vi "Teleop.vi"(10 "Match Info":T1={"Autonomous Elapsed Seconds"=0.0, "TeleOp Elapsed Seconds"=0.0, "Disabled Elapsed Seconds"=0.0, "Visited Autonomous"=FALSE, "Visited TeleOp"=FALSE, "Visited Disabled"=FALSE, "Autonomous Settings"={"Autonomous Style"=enum."Independent", "VI Refnum"=refnum}}, 11 "Call Context":T2) -> ()   [LabVIEW 2018]
doc: "This VI is called for each TeleOp packet received from the DS where the robot is not disabled. It is often used to read from the joysticks and update I/O or to update setpoints for timed control loops. It should complete and return within 20 milliseconds or it may miss DS packets."
uses:
  <vilib>/ptbypt/NI_PtbyPt.lvlib
  <vilib>/addons/control/pid/NI_PID_pid.lvlib
  <vilib>/addons/control/pid/pid.llb/PID Output Rate Limiter (DBL).vi
  <vilib>/Rock Robotics/Network Tables/NT Write Number.vi
  Robot Global Data.vi
  <vilib>/Rock Robotics/Network Tables/NT Write String.vi
  <vilib>/Rock Robotics/Network Tables/NT Write Numeric Array.vi
  <vilib>/Rock Robotics/WPI/DriverStation/WPI_DriverStationMatch Info.ctl
  <vilib>/Rock Robotics/WPI/DriverStation/WPI_DriverStationDerivedRobotMode.ctl
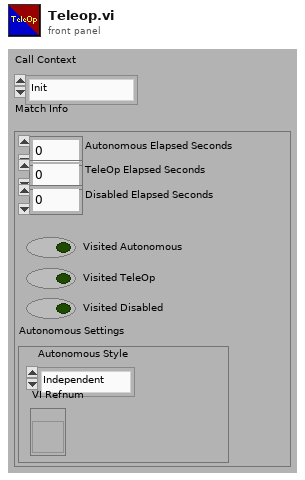
[diagram p1: front panel]
types:
  T1 = typedef "WPI_DriverStationMatch Info.ctl" = cluster{"Autonomous Elapsed Seconds":dbl, "TeleOp Elapsed Seconds":dbl, "Disabled Elapsed Seconds":dbl, "Visited Autonomous":bool, "Visited TeleOp":bool, "Visited Disabled":bool, "Autonomous Settings":cluster{"Autonomous Style":enum16{"Iterative", "Independent"}, "VI Refnum":refnum<vi>}}
  T2 = typedef "WPI_DriverStationDerivedRobotMode.ctl" = enum16{"Init", "Execute", "Stop"}
  T3 = cluster{void, "Filtered x":dbl, "mean":dbl, "output":dbl}
  T4 = typedef "WPI_AnalogChannelDevRef.ctl" = cluster{"DevStatus":errorcluster, "Analog Channel":T5}
  T5 = typedef "FPGA_AIChannel.ctl" = enum8{"AI 0", "AI 1", "AI 2", "AI 3", "AI MXP 0", "AI MXP 1", "AI MXP 2", "AI MXP 3", "Invalid"}
  T6 = typedef "WPI_JoystickDevRef.ctl" = cluster{"Device":T7}
  T7 = typedef "WPI_JoystickDeviceEnum.ctl" = enum16{"USB 0", "USB 1", "USB 2", "USB 3", "USB 4", "USB 5"}
  T8 = typedef "WPI_RobotDriveDevRef.ctl" = cluster{"DevStatus":errorcluster, "Motors[]":T9[], "Square Inputs":bool, "Max Output":dbl}
  T9 = typedef "WPI_MotorControlDeviceRef.ctl" = cluster{"DeviceStatus":errorcluster, "Type":T10, "PWM":cluster{"PWM Channel":T11, "DeadBand":T12}, "CAN":cluster{"Device Number":u8, "SetOutput VI Ref":variant, "GetOutput VI Ref":variant, "Enable VI Ref":variant, "Disable VI Ref":variant, "Data":variant}, "Invert":bool, "DIO PWM":cluster{"PWM \"Enable\" Channel":T11, "DIOChannel":T13, "PWM Rate":dbl}}
  T10 = typedef "WPI_MotorControlType.ctl" = enum16{"PWM", "CAN", "DIO PWM"}
  T11 = typedef "FPGA_DIOPWMChannel.ctl" = enum8{"PWM 0", "PWM 1", "PWM 2", "PWM 3", "PWM 4", "PWM 5", "PWM 6", "PWM 7", "PWM 8", "PWM 9", "PWM MXP 0", "PWM MXP 1", "PWM MXP 2", "PWM MXP 3", "PWM MXP 4", "PWM MXP 5", "PWM MXP 6", "PWM MXP 7", "PWM MXP 8", "PWM MXP 9", "Invalid"}
  T12 = typedef "WPI_PWMDeadband.ctl" = cluster{"Name":string, "maxPositivePwm":i32, "minPositivePwm":i32, "centerPwm":i32, "maxNegativePwm":i32, "minNegativePwm":i32, "angularRange":u16}
  T13 = typedef "FPGA_DIOChannel.ctl" = enum8{"DIO 0", "DIO 1", "DIO 2", "DIO 3", "DIO 4", "DIO 5", "DIO 6", "DIO 7", "DIO 8", "DIO 9", "DIO MXP 0", "DIO MXP 1", "DIO MXP 2", "DIO MXP 3", "DIO MXP 4", "DIO MXP 5", "DIO MXP 6", "DIO MXP 7", "DIO MXP 8", "DIO MXP 9", "DIO MXP 10", "DIO MXP 11", "DIO MXP 12", "DIO MXP 13", "DIO MXP 14", "DIO MXP 15", "SPI Port CS1", "SPI Port CS2", "SPI Port CS3", "SPI Port MISO", "SPI Port MOSI", "Invalid"}
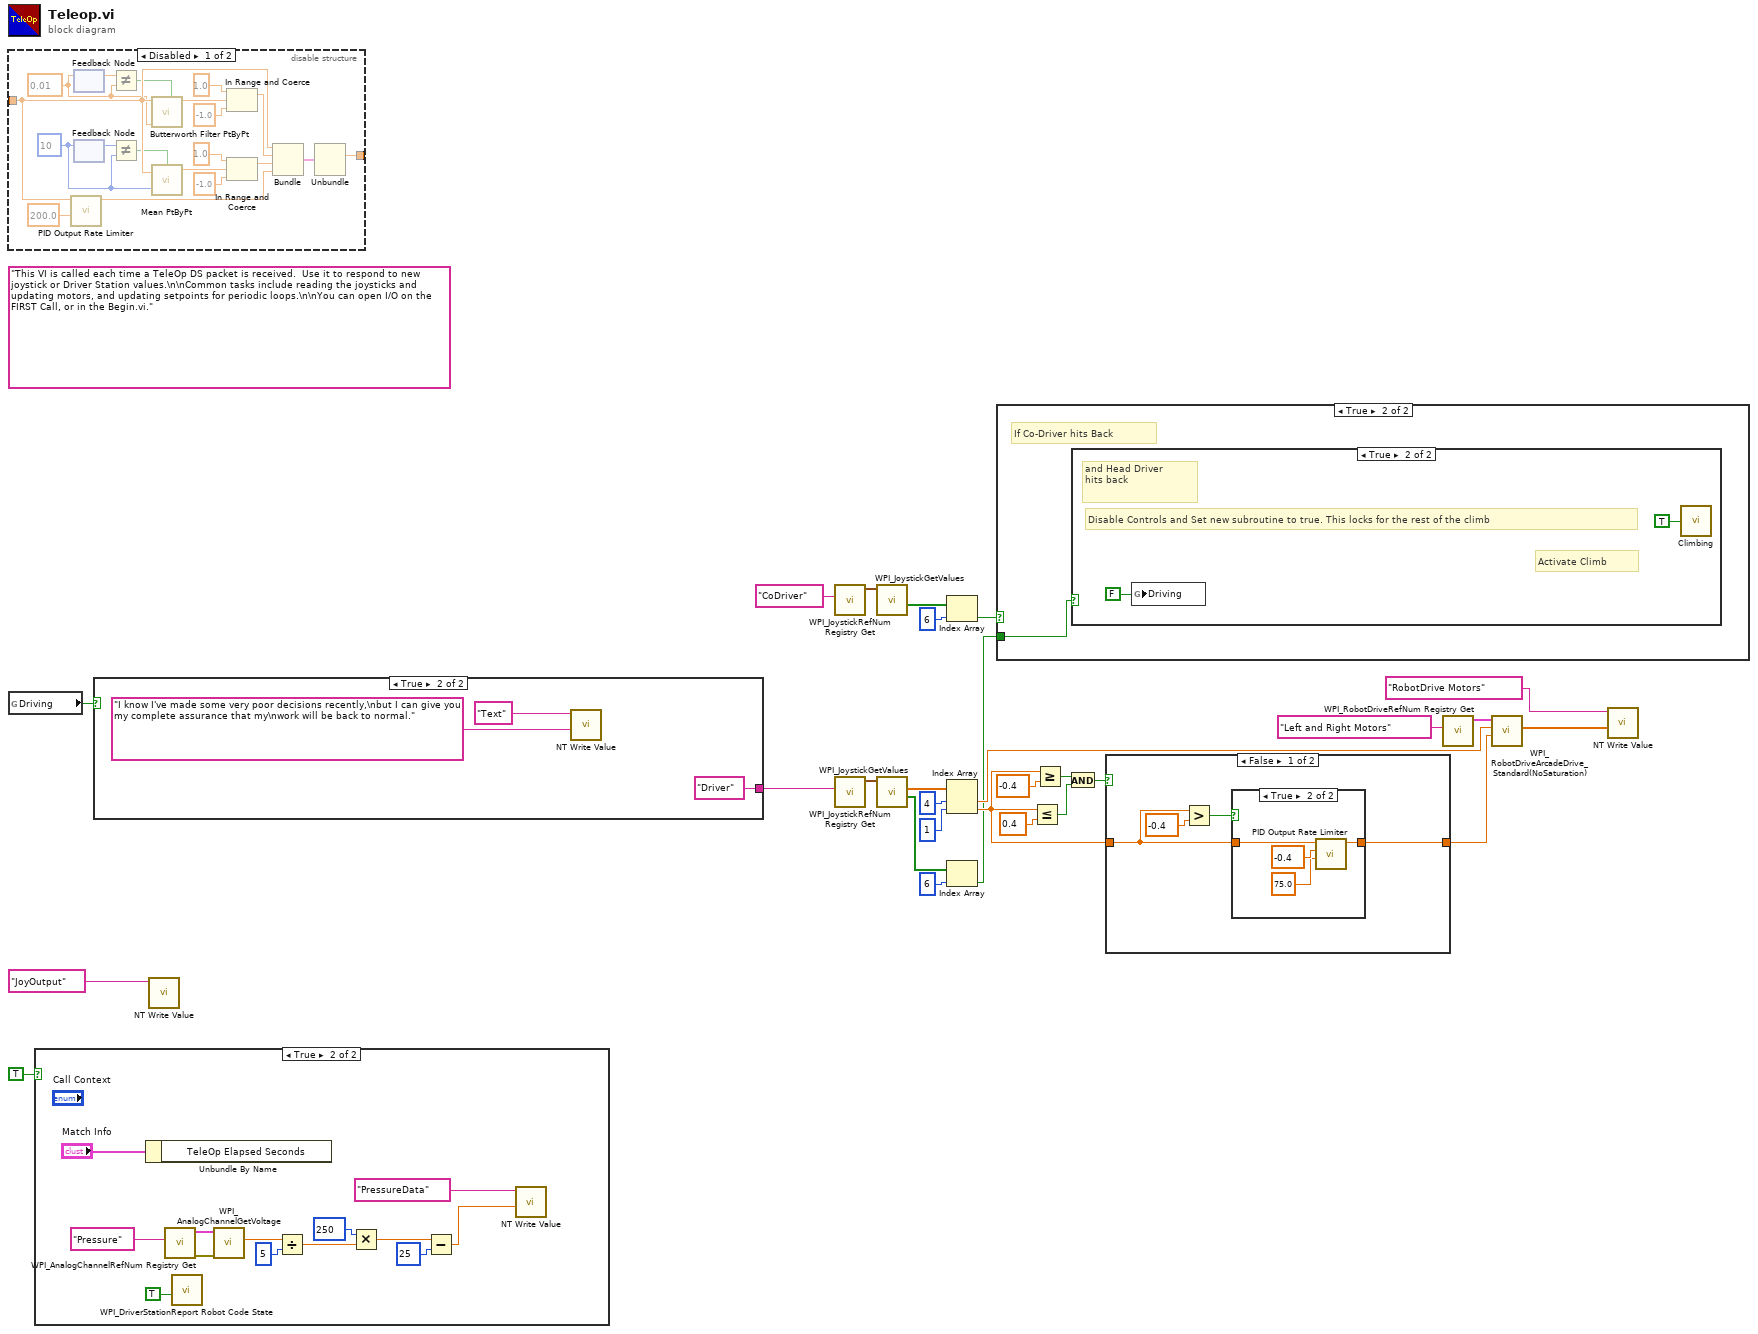
[diagram p0: block diagram]
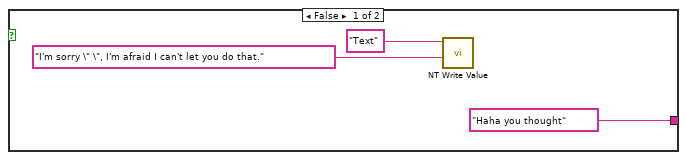
[diagram p5: hidden frame]
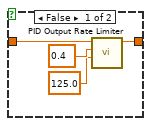
[diagram p6: hidden frame]
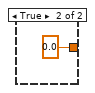
[diagram p7: hidden frame]
diagram:
  (unwired) "This VI is called each time a TeleOp DS packet is received.  Use it to respond to new joystick or Driver Station values.\n\nCommon tasks include reading the joysticks and updating motors, and updating setpoints for periodic loops.\n\nYou can open I/O on the FIRST Call, or in the Begin.vi."
  n1 = disable-structure shown="Disabled" {
    disable-tunnel: _ -> [w47 _]
    disable-tunnel: [w29 _] -> _
    frame Disabled {
      w39 = 10
      w45 = 0.01
      n2 = call-poly <vilib>:"PID Output Rate Limiter.vi"("output rate (EGU/min)"=200.0, "input (controller output)"=w47) -> ("output"=w31:dbl)  [unwired: 6 in, 1 out]
      n3 = feedback #1() -> (w46:dbl)  [unwired: 1 in]
      n4 = feedback-in #1(w45) -> ()
      n5 = feedback #2() -> (w40:i32)  [unwired: 1 in]
      n6 = feedback-in #2(w39) -> ()
      n7 = Not Equal?(x=w46, y=w45) -> (x != y?=w44:bool)
      n8 = Not Equal?(x=w40, y=w39) -> (x != y?=w38:bool)
      n9 = call <vilib>:"Butterworth Filter PtByPt.vi"("initialize"=w44, "low cutoff freq: fl"=w45, "x"=w47) -> ("Filtered x"=w43:dbl)  [unwired: 6 in, 1 out]
      n10 = call <vilib>:"Mean PtByPt.vi"("x"=w47, "sample length"=w39, "initialize"=w38) -> ("mean"=w35:dbl)  [unwired: 1 in, 1 out]
      n11 = In Range and Coerce(upper limit=1.0, x=w43, lower limit=-1.0) -> (coerced(x)=w33:dbl)  [unwired: 1 out]
      n12 = In Range and Coerce(upper limit=1.0, x=w35, lower limit=-1.0) -> (coerced(x)=w32:dbl)  [unwired: 1 out]
      n13 = Bundle(w47, "Filtered x"=w33, "mean"=w32, "output"=w31) -> (w30:T3)  [unwired: 1 in]
      n14 = Unbundle(w30) -> ("Filtered x"=w29:dbl)  [unwired: 3 out]
    }
    frame Enabled {
    }
  }
  n15 = global read "Robot Global Data.vi" "Driving"() -> (w11:bool)
  n16 = case shown="True" TRUE {
    frame False {
    }
    frame True {
      n17 = Unbundle By Name("Match Info") -> ()  [unwired: 1 out]
      n18 = call <vilib>:"WPI_AnalogChannelRefNum Registry Get.vi"("refnum name"="Pressure") -> ("error out"=w57:errorcluster, "AIDeviceRef"=w56:T4)  [unwired: 9 in]
      n19 = call <vilib>:"WPI_DriverStationReport Robot Code State.vi"("TeleOp"=TRUE ("Autonomous")) -> ()  [unwired: 10 in, 1 out]
      n20 = call <vilib>:"WPI_AnalogChannelGetVoltage.vi"("error in (no error)"=w57, "AIDeviceRef"=w56) -> ("Voltage"=w55:dbl)  [unwired: 7 in, 2 out]
      n21 = Divide(x=w55, y=5) -> (x/y=w53:dbl)
      n22 = Multiply(x=250, y=w53) -> (x*y=w50:dbl)
      n23 = Subtract(x=w50, y=25) -> (x-y=w49:dbl)
      n24 = call-poly <vilib>:"NT Write Value.vi"("Numeric"=w49, "Name"="PressureData") -> ()  [unwired: 9 in, 1 out]
    }
  }
  n25 = case shown="True" w11 {
    tunnel: ["Haha you thought" "Driver" ("refnum name")] -> w10
    frame False {
      n26 = call-poly <vilib>:"NT Write Value.vi"("String"="I'm sorry \" \", I'm afraid I can't let you do that.", "Name"="Text") -> ()  [unwired: 9 in, 1 out]
    }
    frame True {
      n27 = call-poly <vilib>:"NT Write Value.vi"("String"="I know I've made some very poor decisions recently,\nbut I can give you my complete assurance that my\nwork will be back to normal.", "Name"="Text") -> ()  [unwired: 9 in, 1 out]
    }
  }
  n28 = call-poly <vilib>:"NT Write Value.vi"("Name"="JoyOutput") -> ()  [unwired: 10 in, 1 out]
  n29 = call <vilib>:"WPI_JoystickRefNum Registry Get.vi"("refnum name"="CoDriver") -> ("JoystickDevRef"=w8:T6)  [unwired: 9 in, 1 out]
  n30 = call <vilib>:"WPI_JoystickRefNum Registry Get.vi"("refnum name"=w10) -> ("JoystickDevRef"=w26:T6)  [unwired: 1 in, 9 out]
  n31 = call <vilib>:"WPI_JoystickGetValues.vi"("JoystickDevRef"=w8) -> ("Buttons"=w7:bool[])  [unwired: 6 in, 4 out]
  n32 = call <vilib>:"WPI_JoystickGetValues.vi"("JoystickDevRef"=w26) -> ("Buttons"=w4:bool[], "Axes"=w25:dbl[])  [unwired: 6 in, 3 out]
  n33 = Index Array(array=w7, index=6) -> (element=w5:bool)
  n34 = Index Array(array=w25, index #1=4, index #2=1) -> (element #1=w14:dbl, element #2=w13:dbl)
  n35 = Index Array(array=w4, index=6) -> (element=w2:bool)
  n36 = case shown="True" w5 {
    tunnel: w2 -> [_ w67]
    frame False {
    }
    frame True {
      # "If Co-Driver hits Back"
      n37 = case shown="True" w67 {
        frame False {
        }
        frame True {
          # "Disable Controls and Set new subroutine to true. This locks for the rest of the climb"
          # "Activate Climb"
          # "and Head Driver\nhits back"
          n38 = global write "Robot Global Data.vi" "Driving"(FALSE ("Driving")) -> ()
          n39 = call "Climbing.vi"("Start Climb?"=TRUE) -> ()
        }
      }
    }
  }
  n40 = Less Or Equal?(x=w13, y=0.4) -> (x <= y?=w17:bool)
  n41 = Greater Or Equal?(x=w13, y=-0.4) -> (x >= y?=w18:bool)
  n42 = And(x=w18, y=w17) -> (x .and. y?=w19:bool)
  n43 = case shown="False" w19 {
    tunnel: [w70 0.0] -> w12
    tunnel: w13 -> [w71 _]
    frame False {
      n44 = Greater?(x=w71, y=-0.4) -> (0:w73:bool)
      n45 = case shown="True" w73 {
        tunnel: w71 -> [w75 w80]
        tunnel: [w74 w79] -> w70
        frame False {
          n46 = call-poly <vilib>:"PID Output Rate Limiter.vi"("output rate (EGU/min)"=125.0, "initial output"=0.4, "input (controller output)"=w75) -> ("output"=w74:dbl)  [unwired: 5 in, 1 out]
        }
        frame True {
          n47 = call-poly <vilib>:"PID Output Rate Limiter.vi"("output rate (EGU/min)"=75.0, "initial output"=-0.4, "input (controller output)"=w80) -> ("output"=w79:dbl)  [unwired: 5 in, 1 out]
        }
      }
    }
    frame True {
    }
  }
  n48 = call <vilib>:"WPI_RobotDriveRefNum Registry Get.vi"("refnum name"="Left and Right Motors") -> ("RobotDriveDevRef"=w27:T8)  [unwired: 1 in, 9 out]
  n49 = call <vilib>:"WPI_RobotDriveArcadeDrive_Standard(NoSaturation).vi"("Y axis value"=w12, "X axis value"=w14, "RobotDriveDevRef"=w27) -> ("Motor Values"=w24:dbl[])  [unwired: 1 in, 7 out]
  n50 = call-poly <vilib>:"NT Write Value.vi"("Numeric Array"=w24, "Name"="RobotDrive Motors") -> ()  [unwired: 9 in, 1 out]
